vi "File_Extract Graphics Files from Folder.vi"(8 "Error":errorcluster, 11 "Graphic Root Folder":path) -> (0 "Error Out":errorcluster, 3 "Array Out":path[](array[path]))   [LabVIEW 2021]
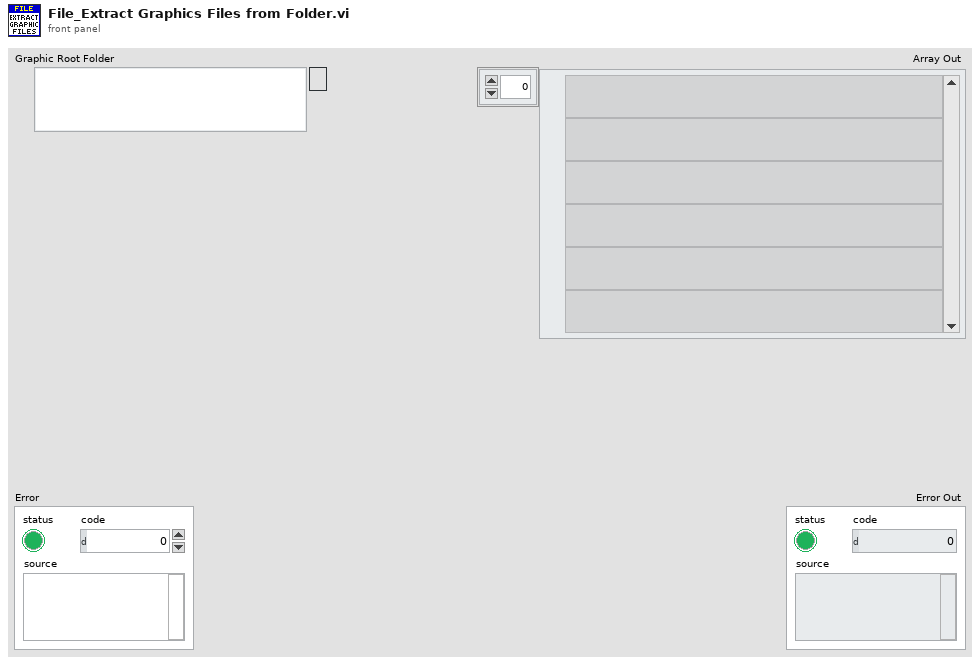
[diagram p1: front panel]
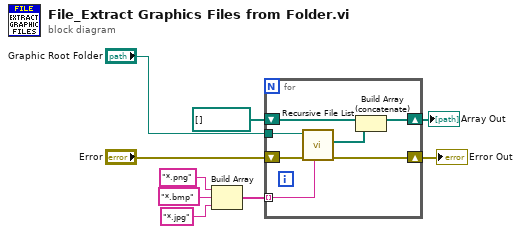
[diagram p0: block diagram]
diagram:
  n1 = Build Array("*.png" ("pattern"), "*.bmp" ("pattern"), "*.jpg" ("pattern")) -> (w4:string[])
  n2 = for {
    tunnel: "Graphic Root Folder" -> [w16]
    shift-right: [w14] -> w2
    shift-left: path[] [] -> [w13]
    tunnel: w4 -> [w15] mode=indexing
    shift-right: [w10] -> w1
    shift-left: "Error" -> [w11]
    n3 = call <vilib>:"Recursive File List.vi"("pattern"=w15, "error in (no error)"=w11, "Folder Path"=w16) -> ("error out"=w10:errorcluster, "All Files in Dir"=w12:path[])  [unwired: 1 in, 6 out]
    n4 = Build Array (concatenate)(w13, w12) -> (w14:path[])
  }
  "Array Out" <- w2
  "Error Out" <- w1
